vi "TemplateMutationMethod.vi"(11 "Version 1":variant) -> (0 "error out":errorcluster, 3 "Version 2":variant)   [LabVIEW 2020]
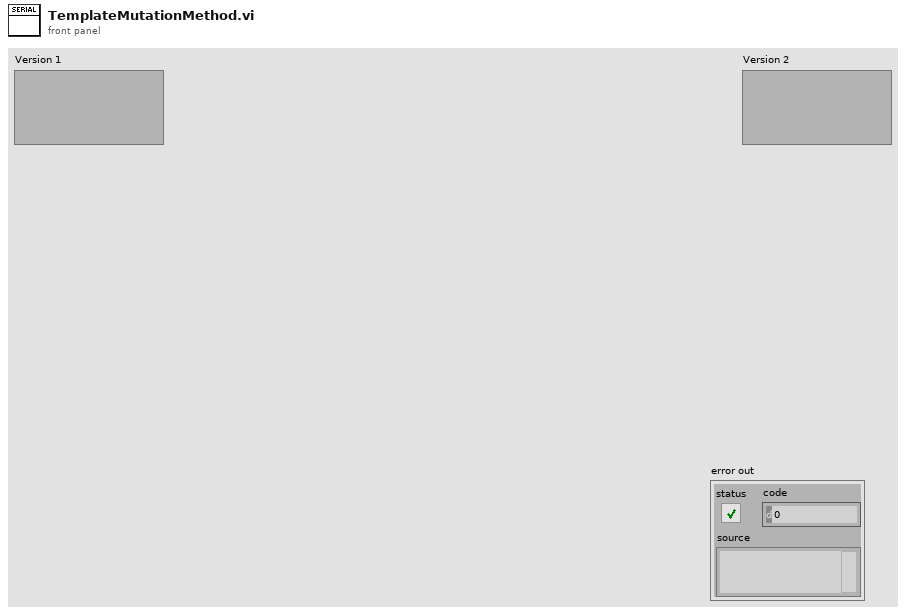
[diagram p1: front panel]
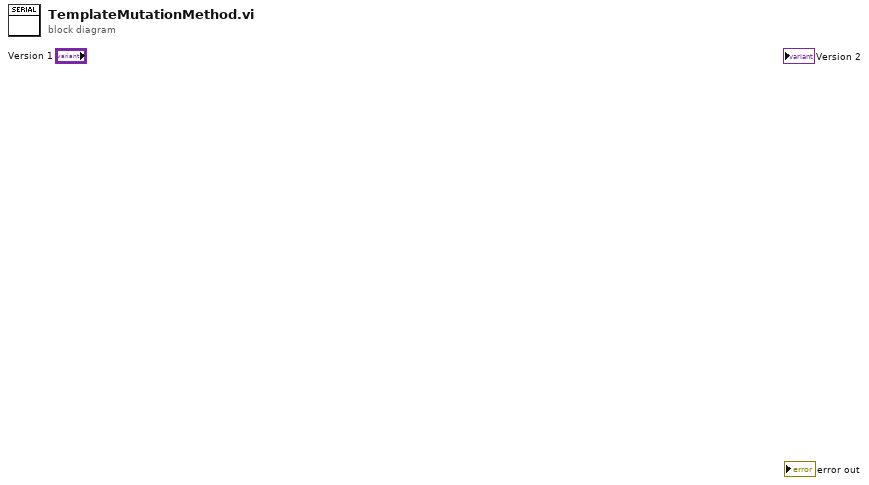
[diagram p0: block diagram]
diagram:
